vi "EMS Shutdown Status.vi"(8 "error in (no error)":errorcluster, 9 "Status":T1, 10 "error":string, 11 "Master Controller in":refnum<class "Master Controller.lvclass">) -> (0 "error out":errorcluster, 3 "Master Controller out":refnum<class "Master Controller.lvclass">)   [LabVIEW 2015, in "Master Controller Core.lvlib" / "Master Controller.lvclass"]
uses:
  Master Controller.lvclass
  SCADA Core/SCADA Abstract Messages/Simple Command Status Msg/Simple Command Status.ctl
  Communications/SCADA Communcations Actor/SCADA Communications/Controls/EMS Message Cluster.ctl
  Master Controller.lvclass/Master Controller.ctl
  Communications/SCADA Communcations Actor/SCADA Communications Messages/Transmit EMS Message Msg/Transmit EMS Message Msg.lvclass/Transmit EMS Message Msg.ctl
  <vilib>/ActorFramework/Message Enqueuer/Message Enqueuer.lvclass/Message Enqueuer.ctl
  <vilib>/ActorFramework/Message Enqueuer/Enqueue.vi
  <vilib>/ActorFramework/Message Priority Queue/Priority Enqueue.vi
  Communications/SCADA Communcations Actor/SCADA Communications Messages/Transmit EMS Message Msg/Transmit EMS Message Msg.lvclass
  Communications/SCADA Communcations Actor/SCADA Communications/SCADA Communications.lvclass
  Utilities/Message Strings.llb/Message String Utilities.lvlib
  SCADA Core/SCADA Abstract Messages/Simple Command Status Msg/Simple Command Status Msg.lvclass
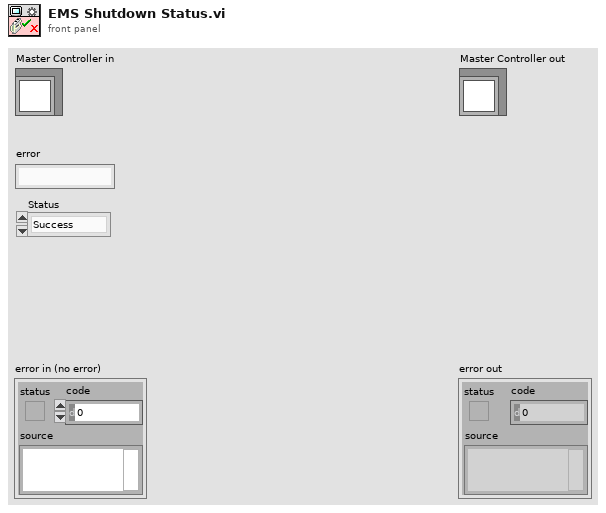
[diagram p1: front panel]
types:
  T1 = typedef "SCADA Core.lvlib/Simple Command Status Msg.lvclass/Simple Command Status.ctl" = enum16{"Success", "Failure"}
  T2 = typedef "SCADA Communcations Actor.lvlib/SCADA Communications.lvclass/EMS Message Cluster.ctl" = cluster{"Name":string, "Content":string}
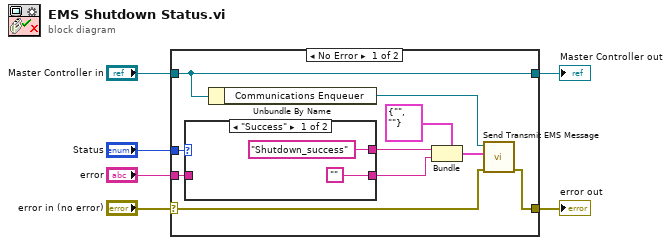
[diagram p0: block diagram]
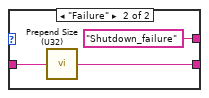
[diagram p2: hidden frame]
diagram:
  n1 = case shown="No Error" "error in (no error)" {
    selector: "error in (no error)" -> [w11 w23]
    tunnel: [w10 w23] -> w5
    tunnel: [w15 w22] -> w3
    tunnel: "Master Controller in" -> [w15 w22]
    tunnel: "error" -> [w8 _]
    tunnel: "Status" -> [w16 _]
    frame No Error {
      n2 = case shown="\"Success\"" w16 {
        tunnel: ["Shutdown_success" ("Name") "Shutdown_failure" ("Name")] -> w9
        tunnel: w8 -> [_ w20]
        tunnel: ["" w19] -> w7
        frame "Success" {
        }
        frame "Failure" {
          n3 = call "Prepend Size (U32).vi"("String in"=w20) -> ("String out"=w19:string)
        }
      }
      n4 = Unbundle By Name(w15) -> ("Communications Enqueuer"=w13:refnum<class "Message Enqueuer.lvclass">)
      n5 = Bundle(cluster=T2 {"Name"="", "Content"=""} ("Message"), "Name"=w9, "Content"=w7) -> (w12:T2)
      n6 = call "Send Transmit EMS Message.vi"("error in (no error)"=w11, "Message"=w12, "Message Enqueuer"=w13) -> ("error out"=w10:errorcluster)  [unwired: 7 in, 1 out]
    }
    frame Error {
    }
  }
  "error out" <- w5
  "Master Controller out" <- w3
